vi "Display GIC 3.vi"(0 "Read GIC":T1={"Real/Sim"=FALSE, "WP Lats and Longs"={"WP Lats"=[], "WP Longs"=[]}, "GPS Time Int"=0.0, "GPS Com Port"="", "Compass Com Port"="", "Prop Com Port"="", "GPS Data"=[], "Compass"=0.0, "LMS Vector"=[], "Vision Vector"=[], "Direction Cmd"=0.0, "Speed Cmd"=0.0, "Time of Last GPS"=0.0, "WP Vector"=[], "WP Number"=0, "Num of WPs"=0, "SW Map"=[], "Obst Lats and Longs"={"Obst Lats"=[], "Obst Longs"=[]}, "Parameters"=[], "Path Cluster"={"Path x nodes"=[], "Path y nodes"=[]}, "     Use ?\nOff       On"=[TRUE, TRUE, FALSE, FALSE]} {"Obst Lats and Longs"."Obst Longs" format="%#_8g"; "Obst Lats and Longs"."Obst Lats" format="%#_8g"}) -> (2 "Display GIC":dbl, 3 "Robot Long":dbl, 4 "Heading":dbl, 6 "Next WP Lat":dbl, 8 "Next WP Long":dbl, 10 "Angle to WP":dbl, 12 "Robot Speed":dbl, 13 "Robot Path Angle":dbl, 14 "WP Number":dbl, 15 "Dist in Meters":dbl)   [LabVIEW 2014]
panel:
  # "GPS"
  # "LMS"
  # "Vision"
  # "Prop"
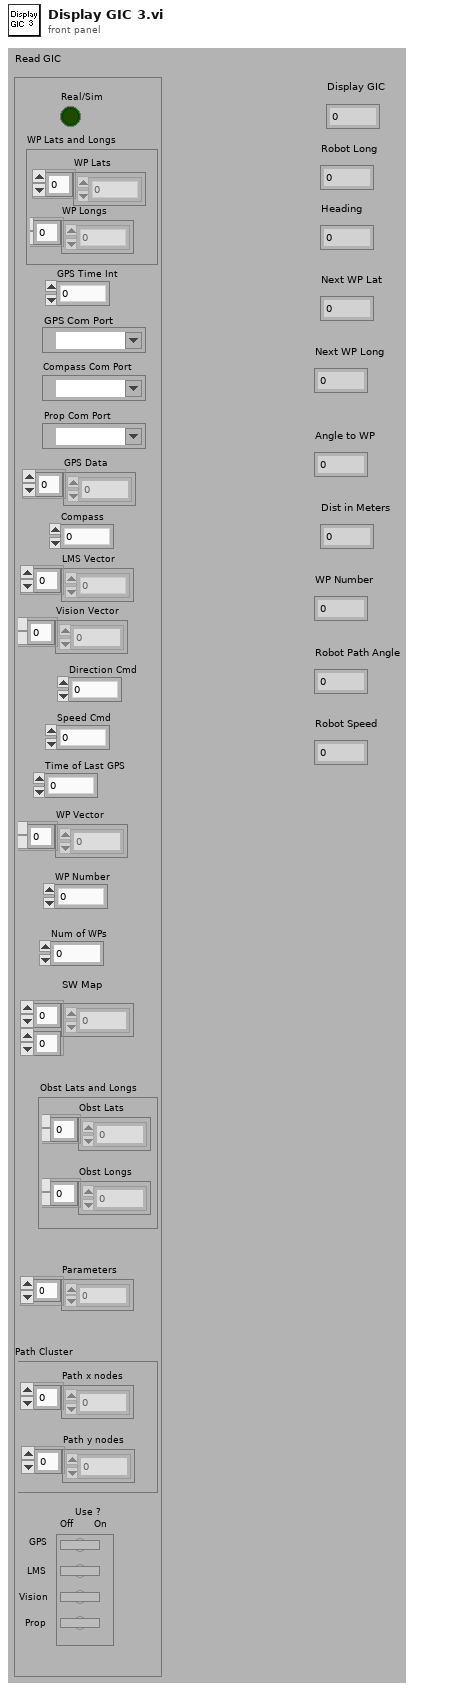
[diagram p1: front panel]
types:
  T1 = cluster{"Real/Sim":bool, "WP Lats and Longs":cluster{"WP Lats":dbl[], "WP Longs":dbl[]}, "GPS Time Int":dbl, "GPS Com Port":refnum<visa-resource-name>, "Compass Com Port":refnum<visa-resource-name>, "Prop Com Port":refnum<visa-resource-name>, "GPS Data":dbl[], "Compass":dbl, "LMS Vector":dbl[], "Vision Vector":dbl[], "Direction Cmd":dbl, "Speed Cmd":dbl, "Time of Last GPS":dbl, "WP Vector":dbl[], "WP Number":i32, "Num of WPs":i16, "SW Map":i32[][], "Obst Lats and Longs":cluster{"Obst Lats":dbl[], "Obst Longs":dbl[]}, "Parameters":dbl[], "Path Cluster":cluster{"Path x nodes":dbl[], "Path y nodes":dbl[]}, "     Use ?\nOff       On":bool[]}
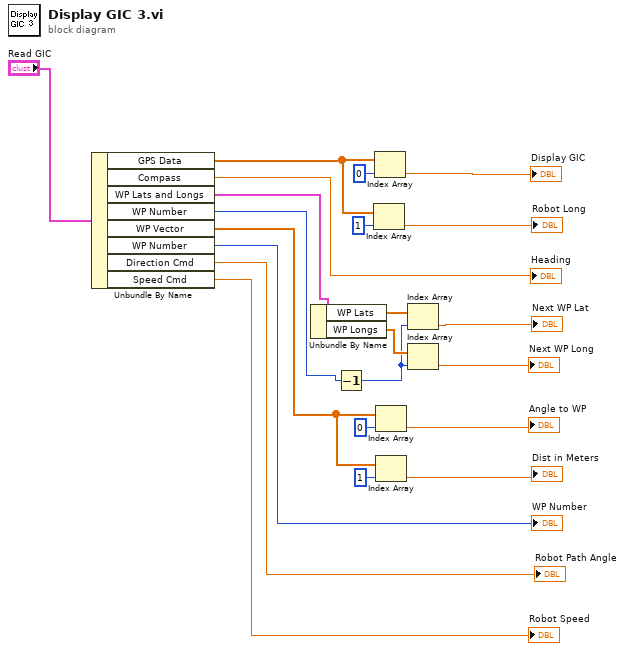
[diagram p0: block diagram]
diagram:
  n1 = Unbundle By Name("Read GIC") -> ("GPS Data"=w21:dbl[], "Compass"=→"Heading":dbl, "WP Lats and Longs"=w16:cluster{"WP Lats":dbl[], "WP Longs":dbl[]}, "WP Number"=w14:i32, "WP Vector"=w7:dbl[], "WP Number"=→"WP Number":i32, "Direction Cmd"=→"Robot Path Angle":dbl, "Speed Cmd"=→"Robot Speed":dbl)
  n2 = Unbundle By Name(w16) -> ("WP Lats"=w15:dbl[], "WP Longs"=w13:dbl[])
  n3 = Decrement(x=w14) -> (x-1=w10:i32)
  n4 = Index Array(array=w21, index=1) -> (element=→"Robot Long":dbl)
  n5 = Index Array(array=w21, index=0) -> (element=→"Display GIC":dbl)
  n6 = Index Array(array=w7, index=0) -> (element=→"Angle to WP":dbl)
  n7 = Index Array(array=w7, index=1) -> (element=→"Dist in Meters":dbl)
  n8 = Index Array(array=w15, index=w10) -> (element=→"Next WP Lat":dbl)
  n9 = Index Array(array=w13, index=w10) -> (element=→"Next WP Long":dbl)
